vi "SaveRunPlan.vi"(8 "error in (no error)":errorcluster, 10 "Path":path, 11 "AutomationContext in":refnum<class "AutomationContext.lvclass">) -> (0 "error out":errorcluster, 3 "AutomationContext out":refnum<class "AutomationContext.lvclass">)   [LabVIEW 2023, in "Automation.lvlib" / "AutomationContext.lvclass"]
uses:
  AutomationContext.lvclass
  AutomationContext.lvclass/AutomationContext.ctl
  b4f4b5c7-678f-4795-9a08-14bbad70606b.vi
  <vilib>/JDP Science/JSONtext/Variant to JSON Text.vi
  <vilib>/JDP Science/JSONtext/LVClass Serializer/JSONtext LVClass Serializer.lvclass
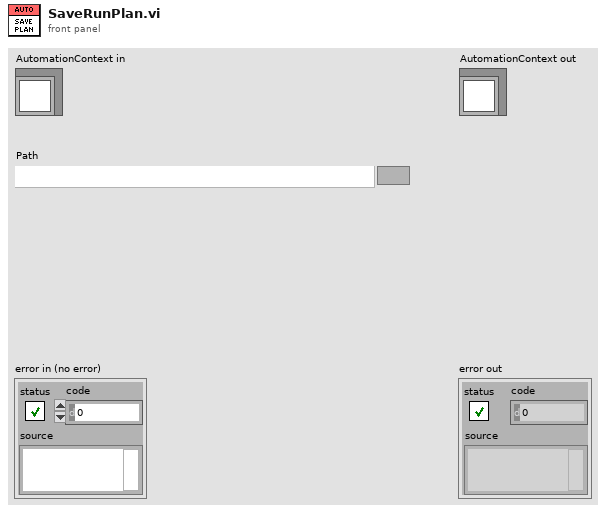
[diagram p1: front panel]
types:
  T1 = typedef "Automation.lvlib/AutomationContext.lvclass/Parallel Block.ctl" = cluster{"Tasks":T2[]}
  T2 = typedef "Automation.lvlib/AutomationContext.lvclass/Automation Intent.ctl" = cluster{"Action":T3, "Parameters":variant, "Correlation ID":u32}
  T3 = typedef "Automation.lvlib/AutomationContext.lvclass/Intent Action.ctl" = enum16{"Next Field", "Next Lane", "Set Power", "Reset Power", "Autofocus", "Start Streaming", "Delay", "Finish Run", "Open Shutter", "Close Shutter"}
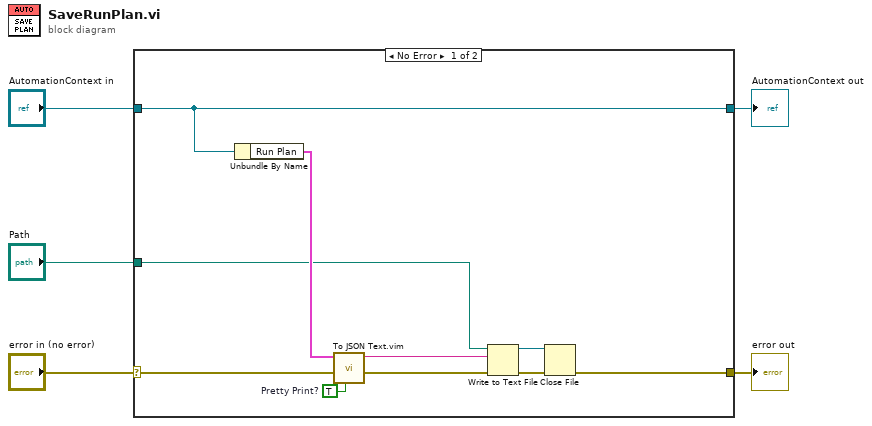
[diagram p0: block diagram]
diagram:
  n1 = case shown="No Error" "error in (no error)" {
    selector: "error in (no error)" -> [w15 w17]
    tunnel: [w10 w17] -> w4
    tunnel: [w14 w16] -> w2
    tunnel: "AutomationContext in" -> [w14 w16]
    tunnel: "Path" -> [w12 _]
    frame No Error {
      w6 = TRUE  # Pretty Print?
      n2 = Unbundle By Name(w14) -> ("Run Plan"=w13:T1[])
      n3 = call "To JSON Text.vim"("Pretty Print?"=w6, "error in (no error)"=w15, "Anything"=w13) -> ("error out"=w8:errorcluster, "<JSON>"=w11:string)  [unwired: 7 in]
      n4 = Write to Text File(file (use dialog)=w12, text=w11, error in=w8) -> (refnum out=w7:refnum<file>, error out=w9:errorcluster)  [unwired: 1 in, 1 out]
      n5 = Close File(refnum=w7, error in=w9) -> (error out=w10:errorcluster)  [unwired: 1 out]
    }
    frame Error {
    }
  }
  "error out" <- w4
  "AutomationContext out" <- w2
